vi "Do Insertion.vi"(8 "error in (no error)":errorcluster, 9 "Insertion Request Time":timestamp, 10 "Viewable":refnum<class "IViewable.lvclass">, 11 "ProtectedSubpanel in":refnum<class "ProtectedSubpanel.lvclass">) -> (0 "error out":errorcluster, 2 "Viewable Out":refnum<class "IViewable.lvclass">, 3 "ProtectedSubpanel out":refnum<class "ProtectedSubpanel.lvclass">)   [LabVIEW 2017, in "IViewable.lvlib" / "ProtectedSubpanel.lvclass"]
uses:
  ProtectedSubpanel.lvclass
  IViewable/IViewable.lvclass
  C:/Program Files (x86)/National Instruments/LabVIEW 2017/vi.lib/ActorFramework/Actor/Actor.lvclass
  ProtectedSubpanel.lvclass/ProtectedSubpanel.ctl
  <vilib>/ActorFramework/Actor/Actor.lvclass/Actor.ctl
  <vilib>/ActorFramework/Message Enqueuer/Message Enqueuer.lvclass/Message Enqueuer.ctl
  IViewable/IViewable.lvclass/IViewable.ctl
  <vilib>/ActorFramework/Message Enqueuer/Message Enqueuer.lvclass
  <vilib>/ActorFramework/Message Enqueuer/Enqueue.vi
  <vilib>/ActorFramework/Actor/Read Self Enqueuer.vi
  <vilib>/ActorFramework/Message Enqueuer/Init from Existing Queue.vi
  IViewable Messages/Removed From Subpanel Msg/Removed From Subpanel Msg.lvclass
  C:/Program Files (x86)/National Instruments/LabVIEW 2017/vi.lib/ActorFramework/Message/Message.lvclass
  <vilib>/ActorFramework/Message Priority Queue/Priority Enqueue.vi
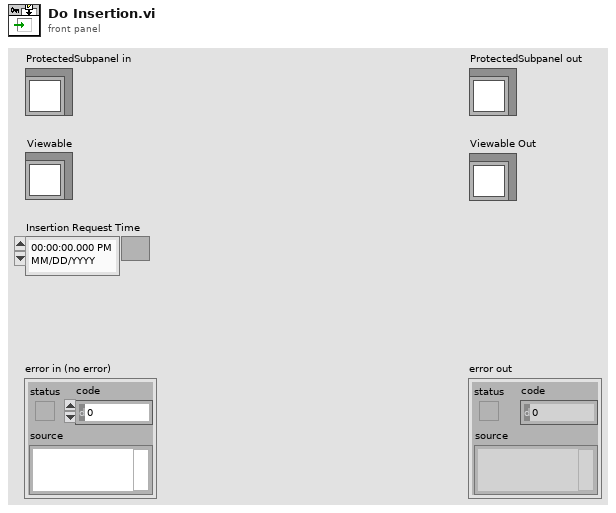
[diagram p1: front panel]
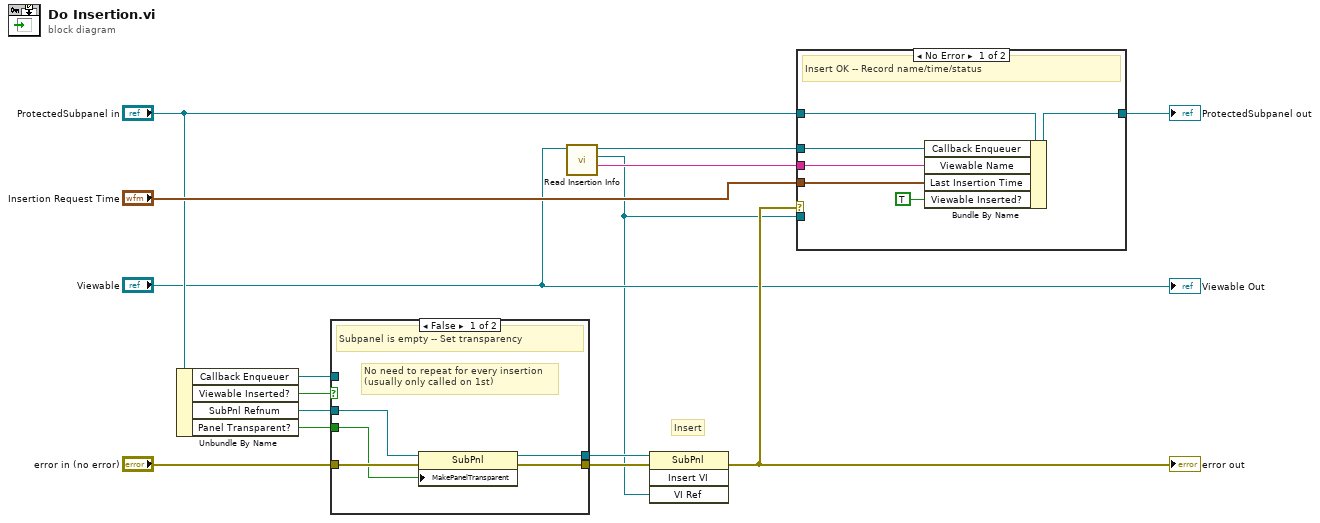
[diagram p0: block diagram]
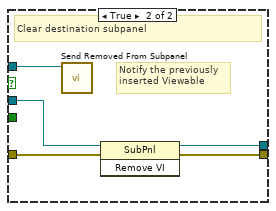
[diagram p2: hidden frame]
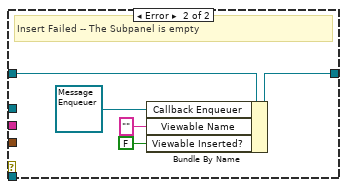
[diagram p3: hidden frame]
diagram:
  # "Insert"
  n1 = Unbundle By Name("ProtectedSubpanel in") -> ("Callback Enqueuer"=w6:refnum<class "Message Enqueuer.lvclass">, "Viewable Inserted?"=w14:bool, "SubPnl Refnum"=w15:refnum<vi>, "Panel Transparent?"=w1:bool)
  n2 = case shown="False" w14 {
    tunnel: w15 -> [w20 w25]
    tunnel: "error in (no error)" -> [w18 w24]
    tunnel: [w19 w23] -> w13
    tunnel: w6 -> [_ w22]
    tunnel: [w17 w21] -> w3
    tunnel: w1 -> [w16 _]
    frame False {
      # "No need to repeat for every insertion\n(usually only called on 1st)"
      # "Subpanel is empty -- Set transparency"
      n3 = property class="SubPnl"(reference=w20, error in=w18, "MakePanelTransparent"=w16) -> (reference out=w19:refnum<vi>, error out=w17:errorcluster)
    }
    frame True {
      # "Notify the previously\ninserted Viewable"
      # "Clear destination subpanel"
      n4 = call "Send Removed From Subpanel.vi"("Message Enqueuer"=w22) -> ()  [unwired: 9 in, 2 out]
      n5 = invoke class="SubPnl" method="Remove VI"(reference=w25, error in=w24) -> (reference out=w23:refnum<vi>, error out=w21:errorcluster)  [unwired: 1 in, 1 out]
    }
  }
  n6 = call "Read Insertion Info.vi"("Viewable in"="Viewable") -> ("Name"=w9:string, "VI Refnum"=w2:refnum<vi>, "Viewable Callback Enqueuer"=w8:refnum<class "Message Enqueuer.lvclass">)  [unwired: 8 in]
  n7 = invoke class="SubPnl" method="Insert VI"(reference=w13, error in=w3, "VI Ref"=w2) -> (error out=w5:errorcluster)  [unwired: 1 in, 3 out]
  "error out" <- w5
  n8 = case shown="No Error" w5 {
    tunnel: [w31 w35] -> w12
    tunnel: "Insertion Request Time" -> [w27 _]
    tunnel: "ProtectedSubpanel in" -> [w30 w36]
    tunnel: w9 -> [w28 _]
    tunnel: w8 -> [w26 _]
    tunnel: w2 -> [_ _]
    frame No Error {
      # "Insert OK -- Record name/time/status"
      n9 = Bundle By Name(cluster=w30, "Callback Enqueuer"=w26, "Viewable Name"=w28, "Last Insertion Time"=w27, "Viewable Inserted?"=TRUE ("View Inserted?")) -> (w31:refnum<class "ProtectedSubpanel.lvclass">)
    }
    frame Error {
      # "Insert Failed -- The Subpanel is empty"
      n10 = Bundle By Name(cluster=w36, "Callback Enqueuer"=refnum<class "Message Enqueuer.lvclass"> refnum ("Viewable Callback Enqueuer"), "Viewable Name"="" ("Inserted View Name"), "Viewable Inserted?"=FALSE) -> (w35:refnum<class "ProtectedSubpanel.lvclass">)
    }
  }
  "ProtectedSubpanel out" <- w12
  "Viewable Out" <- "Viewable"
